vi "VXM Service modularLoop.vi"(6 "Standalone":bool=TRUE, 9 "Motion Cfg File path":path=path "C:/Users/Public/Documents/UCAR/APAR Board Test/SupportFiles/Motion64.ini", 10 "Cfg File path":path=path "C:/Users/Public/Documents/UCAR/APAR Board Test/SupportFiles/APARConfig.ini", 11 "MessageQues":T4) -> ()   [LabVIEW 2018]
doc: "This VI is a simple state machine that has a message que so it can be controlled by external processes.\nIt also has a control with all the messages ques in the calling application that it needs to send messages to.\n\nThe concept is to have many parallel VIs like this one. This VI should be a cohesive process. This could cut down on it's size and complexity.\n\nBolder Software LLC"
uses:
  Support/MessageQue/VXM Main Test App/MultipleMessageQues vxm.ctl
  Support/MessageQue/MessageQue.ctl
  Support/MessageQue/MessageCluster.ctl
  <instrlib>/Velmex VXM/Public/VXM Axis.ctl
  APARMainSubvis/VXM Public API/singleAxisMoveDef.ctl
  APARMainSubvis/VXM Public API/mmWaveAxis.ctl
  Classes/VXMCfg/VXMCfg.lvclass
  Classes/VXMMotionManager/VXMMotionManager.lvclass
  Classes/MotionComm/MotionComm.lvclass
  Classes/sub-systems/sub-systems.lvclass
  Classes/SendMessage/SendMessage.lvclass
  Support/MessageAPI/UIMessage.ctl
  Support/MessageQue/MessageQue.lvlib
  Classes/VSMx2/VXMx2.lvclass
  Classes/aparCfg/aparCfg.lvclass
  <instrlib>/Velmex VXM/Velmex VXM.lvlib
panel:
  out "Position":T1
  out "Axis (1..4)":T3=3 items=["X"=1, "Y"=2, "Z"=3, "T"=4]
  out "i":i32
  out "Command":string
  out "error out":errorcluster
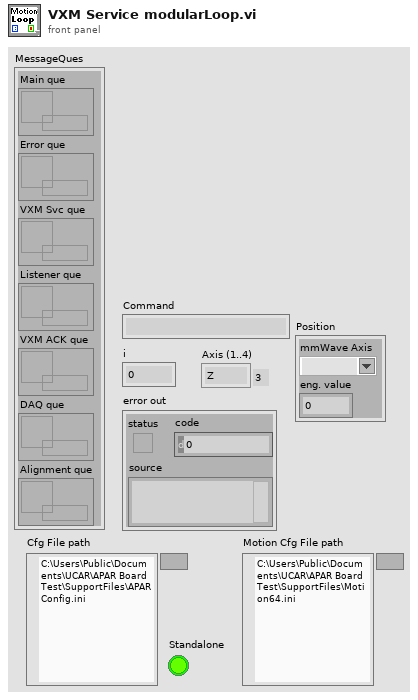
[diagram p1: front panel]
types:
  T1 = typedef "singleAxisMoveDef.ctl" = cluster{"mmWave Axis":T2, "eng. value":dbl}
  T2 = typedef "mmWaveAxis.ctl" = string
  T3 = typedef "Velmex VXM.lvlib/VXM Axis.ctl" = u16
  T4 = typedef "MultipleMessageQues vxm.ctl" = cluster{"Main que":T5, "Error que":T5, "VXM Svc que":T5, "Listener que":T5, "VXM ACK que":T5, "DAQ que":T5, "Alignment que":T5}
  T5 = typedef "MessageQue.lvlib/MessageQue.ctl" = refnum<queue>
  T6 = cluster{"VXMCfg":refnum<class "VXMCfg.lvclass">, "VXMMotionMGr":refnum<class "VXMMotionManager.lvclass">, "Motion":bool, "Motion ACK":refnum<class "MotionComm.lvclass">, "VXM Objects":refnum<class "sub-systems.lvclass">, "UIMsg":refnum<class "SendMessage.lvclass">}
  T7 = typedef "seqConfig.ctl" = cluster{"TempXMLFilePath":path, "Motion":bool}
  T8 = typedef "UIMessage.ctl" = cluster{"EventCode":i32, "Numeric":dbl, "String":string, "Variant":variant}
  T9 = cluster{"Subsystem 1, 2, 3":i32, "Set Home All subsystems":bool}
  T10 = cluster{"Move Type":string, "Positions":T1[], "Position (Antenna or Raster)":i32, "Polarization":u16}
  T11 = typedef "sub-syst.n.ctl" = cluster{"Addr":string, "Enable":bool, "X scale eng./step":dbl, "Y scale eng./step":dbl, "Z scale eng./step":dbl, "T scale eng./step":dbl, "X units":string, "Y units":string, "Z units":string, "T units":string, "X Jog":dbl, "Y Jog":dbl, "Z Jog":dbl, "T Jog":dbl, "X-1 Name":string, "Y-2 Name":string, "Z-3 Name":string, "T-4 Name":string, "VXM (1-4)":i32}
  T12 = cluster{"mmWaveName":string, "Sub-syst":i32, "Axis":string}[]
  T13 = cluster{"mmWave Names":string[], "Positions this subsystem":dbl[]}
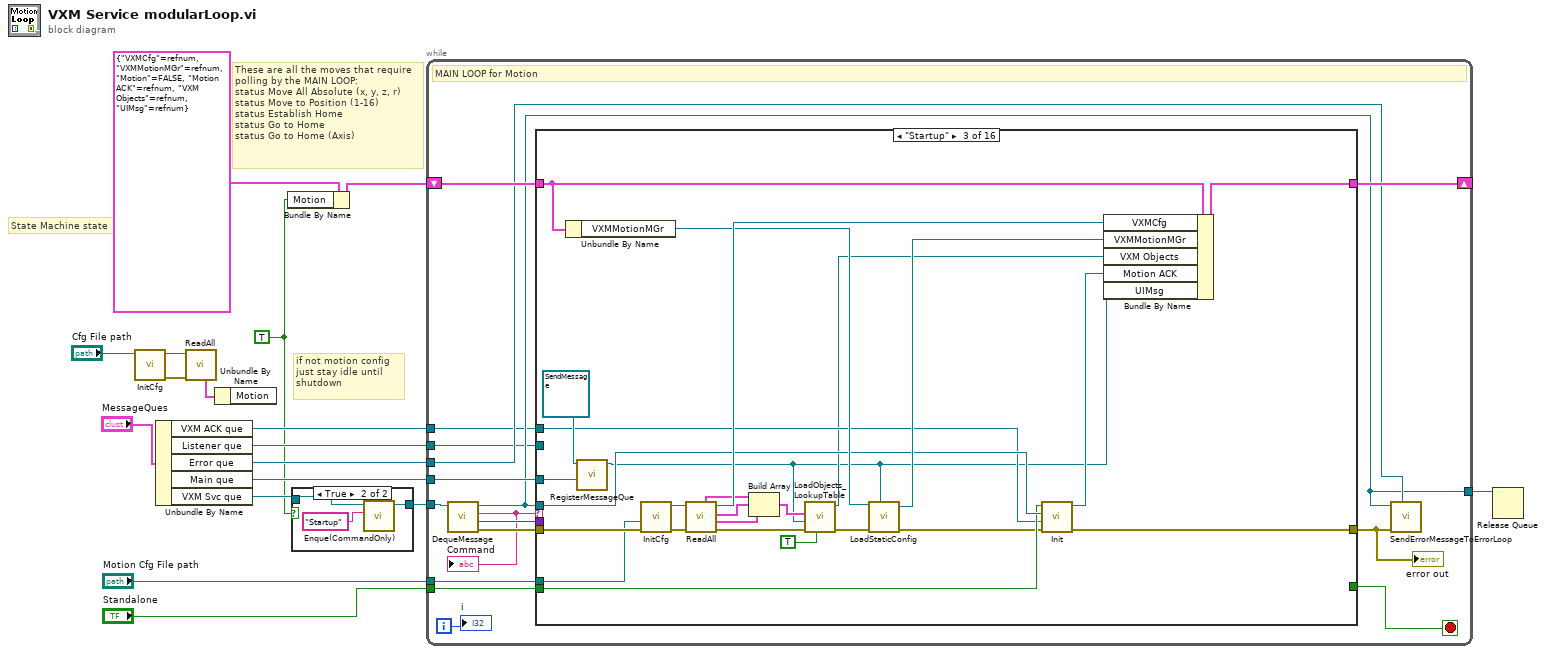
[diagram p0: block diagram]
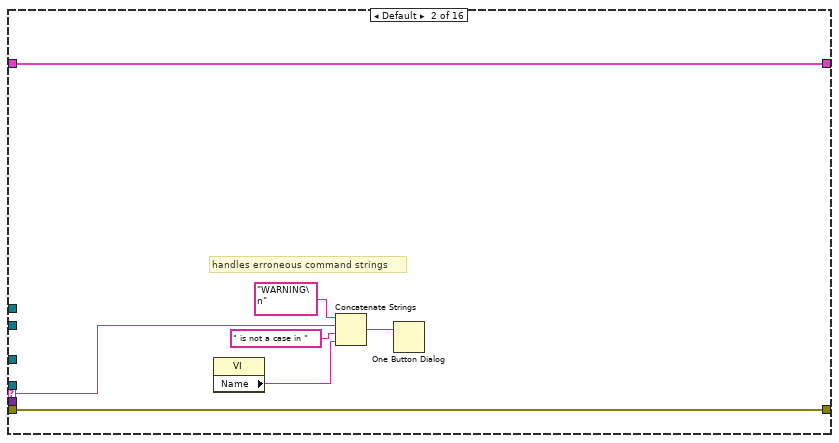
[diagram p4: hidden frame]
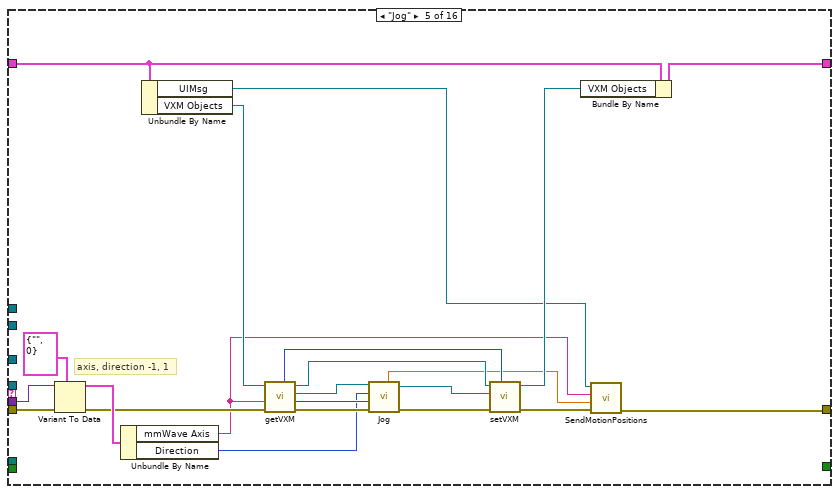
[diagram p6: hidden frame]
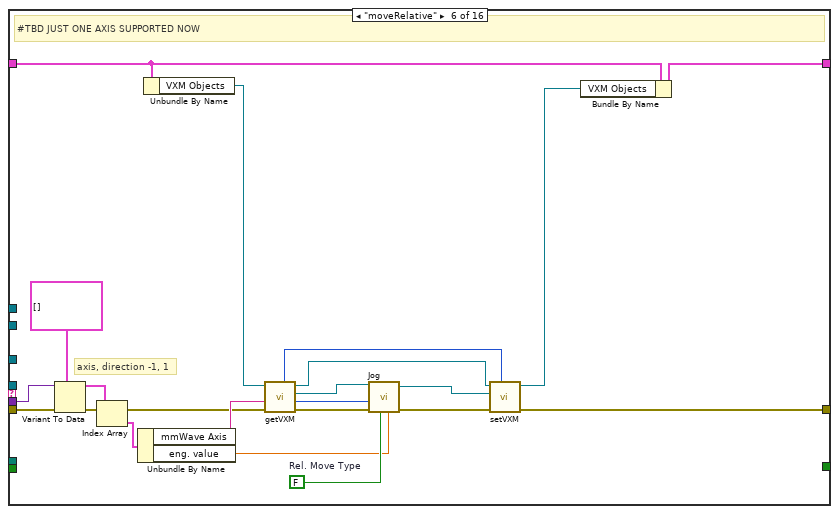
[diagram p7: hidden frame]
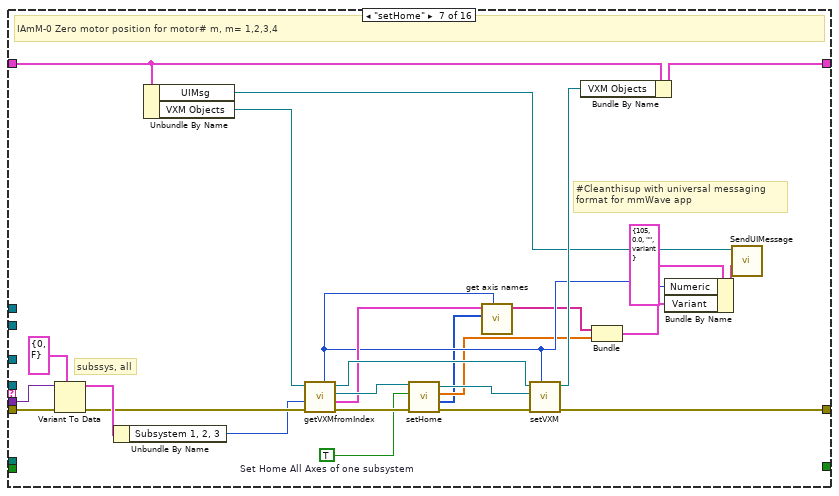
[diagram p8: hidden frame]
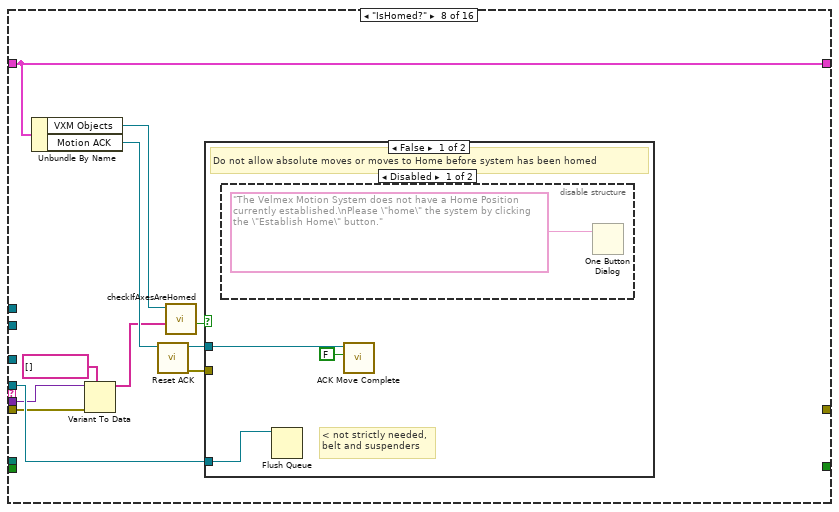
[diagram p9: hidden frame]
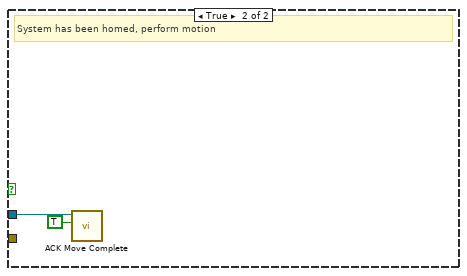
[diagram p11: hidden frame]
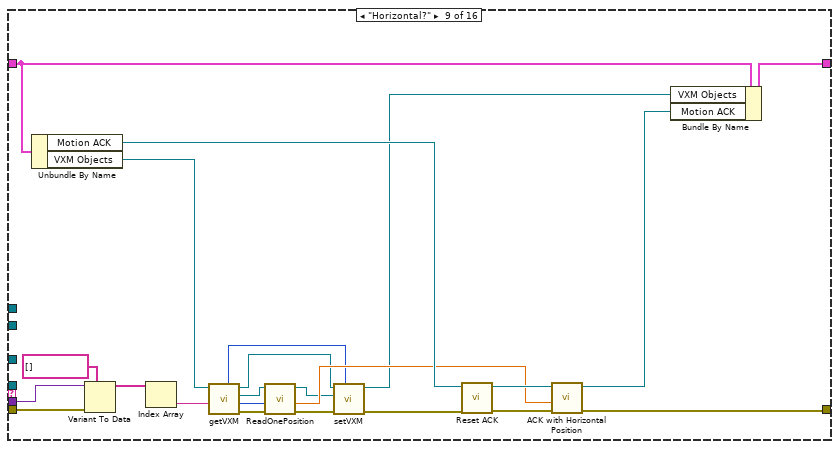
[diagram p12: hidden frame]
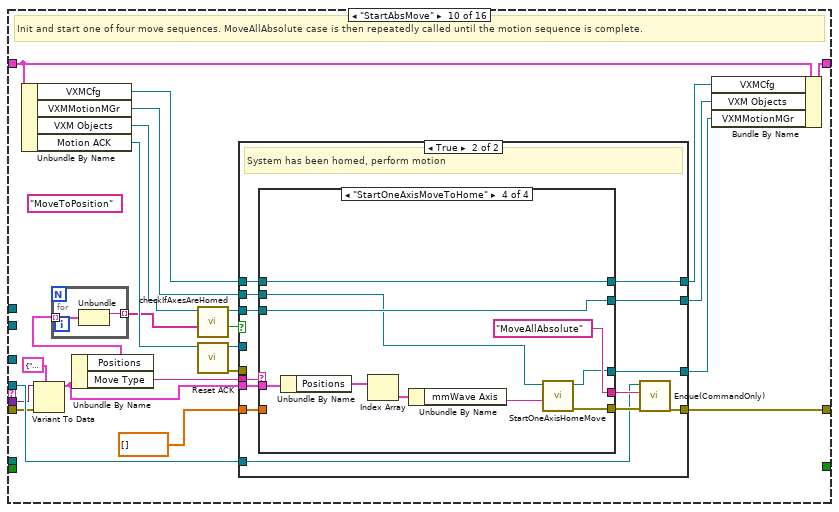
[diagram p13: hidden frame]
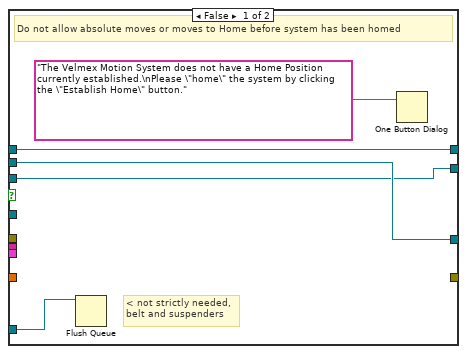
[diagram p14: hidden frame]
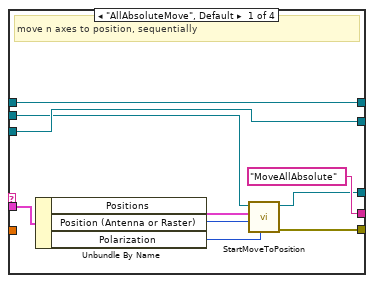
[diagram p15: hidden frame]
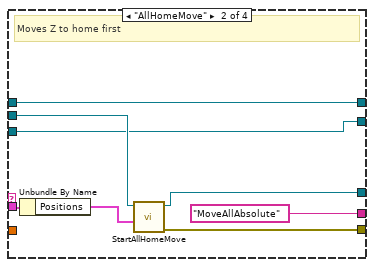
[diagram p16: hidden frame]
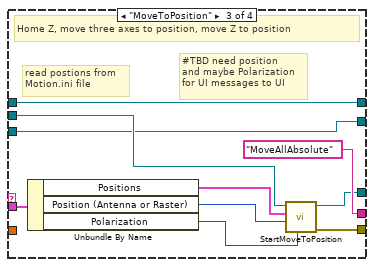
[diagram p17: hidden frame]
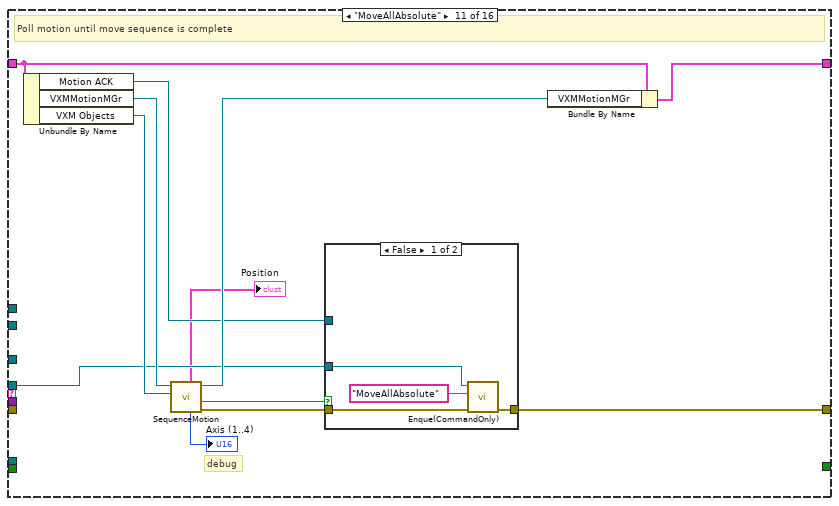
[diagram p18: hidden frame]
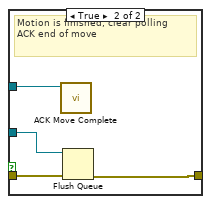
[diagram p19: hidden frame]
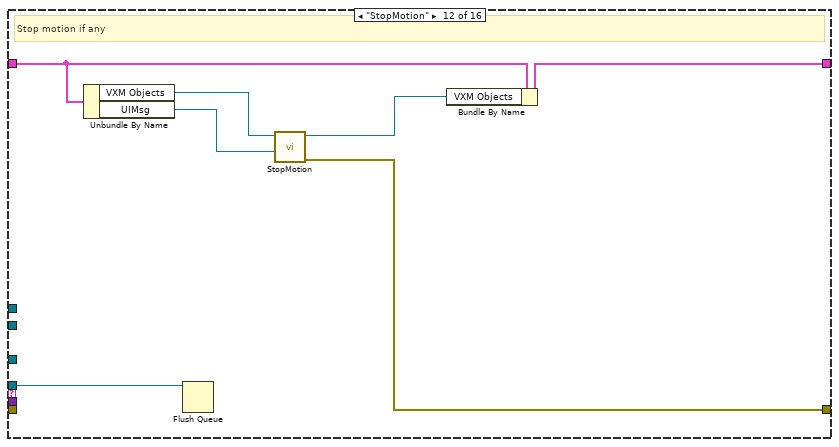
[diagram p20: hidden frame]
diagram:
  w1 = TRUE
  # "if not motion config\njust stay idle until\nshutdown"
  # "These are all the moves that require\npolling by the MAIN LOOP:\nstatus\tMove All Absolute (x, y, z, r)\nstatus\tMove to Position (1-16)\nstatus\tEstablish Home\nstatus\tGo to Home\nstatus\tGo to Home (Axis)"
  # "State Machine state"
  n1 = call "InitCfg.vi"("Cfg File path"="Cfg File path") -> ("error out"=w8:errorcluster, "aparCfg out"=w9:refnum<class "aparCfg.lvclass">)  [unwired: 9 in]
  n2 = Unbundle By Name("MessageQues") -> ("VXM ACK que"=w3:T5, "Listener que"=w11:T5, "Error que"=w15:T5, "Main que"=w16:T5, "VXM Svc que"=w13:T5)
  n3 = call "ReadAll.vi"("error in (no error)"=w8, "aparCfg in"=w9) -> ("SequenceConfig"=w6:T7)  [unwired: 4 in, 5 out]
  n4 = Unbundle By Name(w6) -> ()  [unwired: 1 out]
  n5 = Bundle By Name(cluster=T6 {"VXMCfg"=refnum, "VXMMotionMGr"=refnum, "Motion"=FALSE, "Motion ACK"=refnum, "VXM Objects"=refnum, "UIMsg"=refnum}, "Motion"=w1) -> (w5:T6)
  n6 = case shown="True" w1 {
    tunnel: w13 -> [w18 w21]
    tunnel: [w18 w20] -> w12
    frame False {
    }
    frame True {
      n7 = call "Enque(CommandOnly).vi"("Message Command"="Startup" ("Command"), "Message que"=w21) -> ("Message que out"=w20:T5)  [unwired: 8 in, 1 out]
    }
  }
  n8 = while {
    tunnel: w12 -> [w37]
    tunnel: w16 -> [w36]
    tunnel: w15 -> [w27]
    tunnel: [w26] -> w14
    shift-right: [w32] -> _
    shift-left: w5 -> [w31]
    tunnel: w11 -> [w25]
    tunnel: "Motion Cfg File path" -> [w24]
    tunnel: "Standalone" -> [w23]
    tunnel: w3 -> [w22]
    i -> [w30]
    stop <- w34 stop-if-true
    # "MAIN LOOP for Motion"
    n9 = call "DequeMessage.vi"("Message que"=w37) -> ("error out"=w35:errorcluster, "Message Payload"=w33:variant, "Message Command"=w29:string, "Message que out"=w26:T5)  [unwired: 5 in, 2 out]
    "Command" <- w29
    n10 = case shown="\"Startup\"" w29 {
      selector: w29 -> [_ w40 _ _ _ _ _ _ _ _ _ _ _ _ _ _]
      tunnel: w36 -> [_ _ w63 _ _ _ _ _ _ _ _ _ _ _ _ _]
      tunnel: w26 -> [_ _ w61 _ _ _ _ w147 _ w196 w265 w285 w288 _ _ _]
      tunnel: [_ w45 w47 _ w75 w112 w137 _ w170 w202 w268 w282 _ _ w296 _] -> w28
      tunnel: w35 -> [_ w45 w71 _ w83 w102 w130 w146 w177 w188 _ _ _ _ _ _]
      tunnel: [_ _ _ _ _ _ _ _ _ _ _ _ _ _ _ TRUE] -> w34
      tunnel: w33 -> [_ _ _ _ w82 w101 w129 w145 w176 w183 _ _ _ _ w295 _]
      tunnel: [w38 w44 w68 w72 w93 w113 w138 w143 w173 w200 w272 w286 w289 w293 w297 w301] -> w32
      tunnel: w31 -> [w38 w44 w66 w72 w94 w114 w139 w143 w174 w201 w261 w287 w289 w294 w297 w302]
      tunnel: w25 -> [_ _ _ _ _ _ _ _ _ _ _ _ _ _ _ _]
      tunnel: w24 -> [_ _ w48 _ _ _ _ _ _ _ _ _ _ _ _ _]
      tunnel: w23 -> [_ _ w60 _ _ _ _ _ _ _ _ _ _ _ _ _]
      tunnel: w22 -> [_ _ w59 _ _ _ _ _ _ _ _ _ _ _ _ _]
      frame "idle" {
      }
      frame Default {
        # "handles erroneous command strings"
        n11 = property class="VI"() -> ("Name"=w39:string)  [unwired: 2 in, 2 out]
        n12 = Concatenate Strings("WARNING\n" ("message"), w40, " is not a case in " ("message"), w39) -> (w43:string)
        n13 = One Button Dialog(message=w43) -> ()  [unwired: 1 in, 1 out]
      }
      frame "Startup" {
        n14 = Unbundle By Name(w66) -> ("VXMMotionMGr"=w65:refnum<class "VXMMotionManager.lvclass">)
        n15 = call "RegisterMessageQue.vi"("Message que"=w63, "SendMessage in"=refnum<class "SendMessage.lvclass"> refnum) -> ("SendMessage out"=w46:refnum<class "SendMessage.lvclass">)  [unwired: 8 in, 1 out]
        n16 = call "InitCfg.vi"("error in (no error)"=w71, "Cfg File path"=w48) -> ("error out"=w69:errorcluster, "VXMCfg out"=w70:refnum<class "VXMCfg.lvclass">)  [unwired: 7 in, 1 out]
        n17 = call "ReadAll.vi"("error in (no error)"=w69, "VXMCfg in"=w70) -> ("error out"=w56:errorcluster, "VXM Properties.sub-syst.3"=w53:T11, "VXM Properties.sub-syst.2"=w54:T11, "VXMCfg out"=w67:refnum<class "VXMCfg.lvclass">, "VXM Properties.sub-syst.1"=w55:T11)  [unwired: 5 in]
        n18 = Build Array(w55, w54, w53) -> (w52:T11[])
        n19 = call "LoadObjects_LookupTable.vi"("UIMsgReg."=TRUE, "error in (no error)"=w56, "UIMsg"=w46, "sub-system cfgs"=w52) -> ("error out"=w51:errorcluster, "sub-systems out"=w50:refnum<class "sub-systems.lvclass">)  [unwired: 6 in]
        n20 = call "LoadStaticConfig.vi"("UIMsg"=w46, "error in (no error)"=w51, "VXMMotionManager in"=w65) -> ("error out"=w57:errorcluster, "VXMMotionManager out"=w64:refnum<class "VXMMotionManager.lvclass">)  [unwired: 7 in]
        n21 = call "Init.vi"("error in (no error)"=w57, "VXM ACK que"=w59, "VXM Svc que"=w61, "Standalone"=w60) -> ("error out"=w47:errorcluster, "MotionComm out"=w58:refnum<class "MotionComm.lvclass">)  [unwired: 6 in]
        n22 = Bundle By Name(cluster=w66, "VXMCfg"=w67, "VXMMotionMGr"=w64, "VXM Objects"=w50, "Motion ACK"=w58, "UIMsg"=w46) -> (w68:T6)
      }
      frame "UpdateJogProperties" {
      }
      frame "Jog" {
        # "axis, direction -1, 1"
        n23 = Variant To Data(error in=w83, type=cluster{"mmWave Axis":T2, "Direction":i32} {"mmWave Axis"="", "Direction"=0} ("output cluster"), Variant=w82) -> (data=w91:cluster{"mmWave Axis":T2, "Direction":i32}, error out=w81:errorcluster)
        n24 = Unbundle By Name(w91) -> ("mmWave Axis"=w73:T2, "Direction"=w79:i32)
        n25 = Unbundle By Name(w94) -> ("UIMsg"=w74:refnum<class "SendMessage.lvclass">, "VXM Objects"=w88:refnum<class "sub-systems.lvclass">)
        n26 = call "getVXM.vi"("error in (no error)"=w81, "mmWave Axis Name"=w73, "sub-systems in"=w88) -> ("error out"=w80:errorcluster, "Axis (1..4)"=w84:T3, "VXMx2 out"=w86:refnum<class "VXMx2.lvclass">, "sub-systems out"=w87:refnum<class "sub-systems.lvclass">, "Sub-syst number"=w85:i32)  [unwired: 4 in]
        n27 = call "Jog.vi"("error in (no error)"=w80, "Axis (1..4)"=w84, "Direction -1, 1"=w79, "VXMx2 in"=w86) -> ("error out"=w77:errorcluster, "VXMx2 out"=w89:refnum<class "VXMx2.lvclass">, "Position, eng units"=w78:dbl)  [unwired: 5 in]
        n28 = call "setVXM.vi"("Sub-syst number"=w85, "error in (no error)"=w77, "VXMn"=w89, "sub-systems in"=w87) -> ("error out"=w76:errorcluster, "sub-systems out"=w90:refnum<class "sub-systems.lvclass">)  [unwired: 6 in]
        n29 = Bundle By Name(cluster=w94, "VXM Objects"=w90) -> (w93:T6)
        n30 = call "SendMotionPositions.vi"("error in (no error)"=w76, "Axis Position, eng."=w78, "mmWave Axis Name"=w73, "SendMessage in"=w74) -> ("error out"=w75:errorcluster)  [unwired: 6 in, 1 out]
      }
      frame "moveRelative" {
        w98 = FALSE  # Rel. Move Type
        # "axis, direction -1, 1"
        # "#TBD JUST ONE AXIS SUPPORTED NOW"
        n31 = Variant To Data(error in=w102, type=T1[] [] ("Moves"), Variant=w101) -> (data=w111:T1[], error out=w100:errorcluster)
        n32 = Index Array(array=w111) -> (element=w95:T1)  [unwired: 1 in]
        n33 = Unbundle By Name(w95) -> ("mmWave Axis"=w108:T2, "eng. value"=w97:dbl)
        n34 = Unbundle By Name(w114) -> ("VXM Objects"=w107:refnum<class "sub-systems.lvclass">)
        n35 = call "getVXM.vi"("error in (no error)"=w100, "mmWave Axis Name"=w108, "sub-systems in"=w107) -> ("error out"=w99:errorcluster, "Axis (1..4)"=w103:T3, "VXMx2 out"=w105:refnum<class "VXMx2.lvclass">, "sub-systems out"=w106:refnum<class "sub-systems.lvclass">, "Sub-syst number"=w104:i32)  [unwired: 4 in]
        n36 = call "Jog.vi"("One Axis Rel Distanz mm"=w97, "Rel. Move Type"=w98, "error in (no error)"=w99, "Axis (1..4)"=w103, "VXMx2 in"=w105) -> ("error out"=w112:errorcluster, "VXMx2 out"=w109:refnum<class "VXMx2.lvclass">)  [unwired: 4 in, 1 out]
        n37 = call "setVXM.vi"("Sub-syst number"=w104, "VXMn"=w109, "sub-systems in"=w106) -> ("sub-systems out"=w110:refnum<class "sub-systems.lvclass">)  [unwired: 7 in, 1 out]
        n38 = Bundle By Name(cluster=w114, "VXM Objects"=w110) -> (w113:T6)
      }
      frame "setHome" {
        w124 = TRUE  # Set Home All Axes of one subsystem
        # "#Cleanthisup with universal messaging \nformat for mmWave app"
        # "subssys, all"
        # "IAmM-0 Zero motor position for motor# m, m= 1,2,3,4"
        n39 = Variant To Data(error in=w130, type=T9 {"Subsystem 1, 2, 3"=0, "Set Home All subsystems"=FALSE} ("output cluster"), Variant=w129) -> (data=w136:T9, error out=w128:errorcluster)
        n40 = Unbundle By Name(w136) -> ("Subsystem 1, 2, 3"=w125:i32)
        n41 = Unbundle By Name(w139) -> ("UIMsg"=w121:refnum<class "SendMessage.lvclass">, "VXM Objects"=w133:refnum<class "sub-systems.lvclass">)
        n42 = call "getVXMfromIndex.vi"("error in (no error)"=w128, "Subsystem 1, 2, 3"=w125, "sub-systems in"=w133) -> ("error out"=w127:errorcluster, "All Axes this subsystem"=w120:T12, "VXMx2 out"=w131:refnum<class "VXMx2.lvclass">, "sub-systems out"=w132:refnum<class "sub-systems.lvclass">, "Sub-syst number"=w119:i32)  [unwired: 4 in]
        n43 = call "setHome.vi"("error in (no error)"=w127, "Set Home All Axes"=w124, "VXMx2 in"=w131) -> ("error out"=w137:errorcluster, "Axes"=w115:T3[], "Positions this subsystem"=w117:dbl[], "VXMx2 out"=w134:refnum<class "VXMx2.lvclass">)  [unwired: 5 in]
        n44 = call "get axis names.vi"("Subsystem 1, 2, 3"=w119, "Axes"=w115, "Lookup Table"=w120) -> ("mmWave Names"=w118:string[])  [unwired: 8 in]
        n45 = call "setVXM.vi"("Sub-syst number"=w119, "VXMn"=w134, "sub-systems in"=w132) -> ("sub-systems out"=w135:refnum<class "sub-systems.lvclass">)  [unwired: 7 in, 1 out]
        n46 = Bundle By Name(cluster=w139, "VXM Objects"=w135) -> (w138:T6)
        n47 = Bundle("mmWave Names"=w118, "Positions this subsystem"=w117) -> (w116:T13)  [unwired: 1 in]
        n48 = Bundle By Name(cluster=T8 {"EventCode"=105, "Numeric"=0.0, "String"="", "Variant"=variant} ("UIMsg"), "Numeric"=w119, "Variant"=w116) -> (w122:T8)
        n49 = call-dynamic "SendUIMessage.vi"("UIMsg"=w122, "SendMessage in"=w121) -> ()  [unwired: 8 in, 2 out]
      }
      frame "IsHomed?" {
        n50 = Unbundle By Name(w143) -> ("VXM Objects"=w142:refnum<class "sub-systems.lvclass">, "Motion ACK"=w150:refnum<class "MotionComm.lvclass">)
        n51 = Variant To Data(error in=w146, type=T2[] [] ("check these axes homed"), Variant=w145) -> (data=w141:T2[])  [unwired: 1 out]
        n52 = call "Reset ACK.vi"("MotionComm in"=w150) -> ("error out"=w149:errorcluster, "MotionComm out"=w148:refnum<class "MotionComm.lvclass">)  [unwired: 9 in]
        n53 = call "checkIfAxesAreHomed.vi"("check these axes homed"=w141, "sub-systems in"=w142) -> ("Homed=T"=w140:bool)  [unwired: 7 in, 2 out]
        n54 = case shown="False" w140 {
          tunnel: w147 -> [w153 _]
          tunnel: w149 -> [_ _]
          tunnel: w148 -> [w152 w155]
          frame False {
            # "< not strictly needed,\nbelt and suspenders"
            # "Do not allow absolute moves or moves to Home before system has been homed"
            n55 = disable-structure shown="Disabled" {
              frame Disabled {
                n56 = One Button Dialog(message="The Velmex Motion System does not have a Home Position currently established.\nPlease \"home\" the system by clicking the \"Establish Home\" button.") -> ()  [unwired: 1 in, 1 out]
              }
              frame Enabled {
              }
            }
            n57 = Flush Queue(queue=w153) -> ()  [unwired: 1 in, 3 out]
            n58 = call "ACK Move Complete.vi"("Motion ACK = True"=FALSE, "MotionComm in"=w152) -> ()  [unwired: 8 in, 2 out]
          }
          frame True {
            # "System has been homed, perform motion"
            n59 = call "ACK Move Complete.vi"("Motion ACK = True"=TRUE, "MotionComm in"=w155) -> ()  [unwired: 8 in, 2 out]
          }
        }
      }
      frame "Horizontal?" {
        n60 = Unbundle By Name(w174) -> ("Motion ACK"=w179:refnum<class "MotionComm.lvclass">, "VXM Objects"=w168:refnum<class "sub-systems.lvclass">)
        n61 = Variant To Data(error in=w177, type=T2[] [] ("check these axes homed"), Variant=w176) -> (data=w169:T2[])  [unwired: 1 out]
        n62 = Index Array(array=w169) -> (element=w167:T2)  [unwired: 1 in]
        n63 = call "getVXM.vi"("mmWave Axis Name"=w167, "sub-systems in"=w168) -> ("error out"=w166:errorcluster, "Axis (1..4)"=w164:T3, "VXMx2 out"=w165:refnum<class "VXMx2.lvclass">, "sub-systems out"=w159:refnum<class "sub-systems.lvclass">, "Sub-syst number"=w160:i32)  [unwired: 5 in]
        n64 = call "ReadOnePosition.vi"("error in (no error)"=w166, "Axis (1..4)"=w164, "VXMx2 in"=w165) -> ("error out"=w162:errorcluster, "Position, eng units"=w163:dbl, "VXMx2 out"=w158:refnum<class "VXMx2.lvclass">)  [unwired: 6 in]
        n65 = call "setVXM.vi"("Sub-syst number"=w160, "error in (no error)"=w162, "VXMn"=w158, "sub-systems in"=w159) -> ("error out"=w161:errorcluster, "sub-systems out"=w157:refnum<class "sub-systems.lvclass">)  [unwired: 6 in]
        n66 = call "Reset ACK.vi"("error in (no error)"=w161, "MotionComm in"=w179) -> ("error out"=w171:errorcluster, "MotionComm out"=w178:refnum<class "MotionComm.lvclass">)  [unwired: 8 in]
        n67 = call "ACK with Horizontal Position.vi"("error in (no error)"=w171, "Horizontal position, degrees"=w163, "MotionComm in"=w178) -> ("error out"=w170:errorcluster, "MotionComm out"=w172:refnum<class "MotionComm.lvclass">)  [unwired: 7 in]
        n68 = Bundle By Name(cluster=w174, "VXM Objects"=w157, "Motion ACK"=w172) -> (w173:T6)
      }
      frame "StartAbsMove" {
        (unwired) "MoveToPosition" ("MoveType")
        # "Init and start one of four move sequences. MoveAllAbsolute case is then repeatedly called until the motion sequence is complete."
        n69 = Unbundle By Name(w201) -> ("VXMCfg"=w195:refnum<class "VXMCfg.lvclass">, "VXMMotionMGr"=w199:refnum<class "VXMMotionManager.lvclass">, "VXM Objects"=w180:refnum<class "sub-systems.lvclass">, "Motion ACK"=w193:refnum<class "MotionComm.lvclass">)
        n70 = Variant To Data(error in=w188, type=T10 {"Move Type"="OneAxisHomeMove", "Positions"=[], "Position (Antenna or Raster)"=0, "Polarization"=0} ("Move-Abs"), Variant=w183) -> (data=w185:T10)  [unwired: 1 out]
        n71 = Unbundle By Name(w185) -> ("Positions"=w182:T1[], "Move Type"=w186:string)
        n72 = for {
          tunnel: w182 -> [w204] mode=indexing
          tunnel: [w203] -> w181 mode=indexing
          n73 = Unbundle(w204) -> ("mmWave Axis"=w203:T2)  [unwired: 1 out]
        }
        n74 = call "checkIfAxesAreHomed.vi"("check these axes homed"=w181, "sub-systems in"=w180) -> ("Homed=T"=w189:bool, "sub-systems out"=w190:refnum<class "sub-systems.lvclass">)  [unwired: 7 in, 1 out]
        n75 = call "Reset ACK.vi"("MotionComm in"=w193) -> ("error out"=w192:errorcluster, "MotionComm out"=w191:refnum<class "MotionComm.lvclass">)  [unwired: 9 in]
        n76 = case shown="True" w189 {
          tunnel: [_ w222] -> w202
          tunnel: w186 -> [_ w221]
          tunnel: w199 -> [w209 w220]
          tunnel: dbl[] [] ("Move Params") -> [_ w219]
          tunnel: [w209 w216] -> w197
          tunnel: w190 -> [w205 w215]
          tunnel: w196 -> [w207 w214]
          tunnel: w195 -> [w206 w213]
          tunnel: [w206 w212] -> w194
          tunnel: w192 -> [_ _]
          tunnel: w191 -> [_ _]
          tunnel: w185 -> [_ w211]
          tunnel: [w205 w210] -> w187
          frame False {
            # "< not strictly needed,\nbelt and suspenders"
            # "Do not allow absolute moves or moves to Home before system has been homed"
            n77 = Flush Queue(queue=w207) -> ()  [unwired: 1 in, 3 out]
            n78 = One Button Dialog(message="The Velmex Motion System does not have a Home Position currently established.\nPlease \"home\" the system by clicking the \"Establish Home\" button.") -> ()  [unwired: 1 in, 1 out]
          }
          frame True {
            # "System has been homed, perform motion"
            n79 = case shown="\"StartOneAxisMoveToHome\"" w221 {
              tunnel: w220 -> [w226 w240 w246 w254]
              tunnel: w219 -> [_ _ _ _]
              tunnel: ["MoveAllAbsolute" ("Command") "MoveAllAbsolute" ("Command") "MoveAllAbsolute" ("Command") "MoveAllAbsolute" ("Command")] -> w218
              tunnel: [w229 w238 w249 w256] -> w217
              tunnel: w215 -> [w230 w235 w245 w258]
              tunnel: [w228 w237 w248 w255] -> w216
              tunnel: w213 -> [w231 w236 w247 w259]
              tunnel: [w231 w236 w247 w259] -> w212
              tunnel: w211 -> [w227 w234 w244 w257]
              tunnel: [w230 w235 w245 w258] -> w210
              frame "AllAbsoluteMove", Default {
                # "move n axes to position, sequentially"
                n80 = Unbundle By Name(w227) -> ("Positions"=w223:T1[], "Position (Antenna or Raster)"=w225:i32, "Polarization"=w224:u16)
                n81 = call "StartMoveToPosition.vi"("Polarization"=w224, "Position (Antenna or Raster)"=w225, "Positions"=w223, "VXMMotionManager in"=w226) -> ("error out"=w229:errorcluster, "VXMMotionManager out"=w228:refnum<class "VXMMotionManager.lvclass">)  [unwired: 6 in]
              }
              frame "AllHomeMove" {
                # "Moves Z to home first"
                n82 = Unbundle By Name(w234) -> ("Positions"=w233:T1[])
                n83 = call "StartAllHomeMove.vi"("Positions to home"=w233, "VXMMotionManager in"=w240) -> ("error out"=w238:errorcluster, "VXMMotionManager out"=w237:refnum<class "VXMMotionManager.lvclass">)  [unwired: 8 in]
              }
              frame "MoveToPosition" {
                # "#TBD need position\nand maybe Polarization\nfor UI messages to UI"
                # "read postions from \nMotion.ini file"
                # "Home Z, move three axes to position, move Z to position"
                n84 = Unbundle By Name(w244) -> ("Positions"=w243:T1[], "Position (Antenna or Raster)"=w242:i32, "Polarization"=w241:u16)
                n85 = call "StartMoveToPosition.vi"("Polarization"=w241, "Position (Antenna or Raster)"=w242, "Positions"=w243, "VXMMotionManager in"=w246) -> ("error out"=w249:errorcluster, "VXMMotionManager out"=w248:refnum<class "VXMMotionManager.lvclass">)  [unwired: 6 in]
              }
              frame "StartOneAxisMoveToHome" {
                n86 = Unbundle By Name(w257) -> ("Positions"=w253:T1[])
                n87 = Index Array(array=w253) -> (element=w252:T1)  [unwired: 1 in]
                n88 = Unbundle By Name(w252) -> ("mmWave Axis"=w251:T2)
                n89 = call "StartOneAxisHomeMove.vi"("mmWave Axis to Home"=w251, "VXMMotionManager in"=w254) -> ("error out"=w256:errorcluster, "VXMMotionManager out"=w255:refnum<class "VXMMotionManager.lvclass">)  [unwired: 8 in]
              }
            }
            n90 = call "Enque(CommandOnly).vi"("error in"=w217, "Message Command"=w218, "Message que"=w214) -> ("error out"=w222:errorcluster)  [unwired: 7 in, 1 out]
          }
        }
        n91 = Bundle By Name(cluster=w201, "VXMCfg"=w194, "VXM Objects"=w187, "VXMMotionMGr"=w197) -> (w200:T6)
      }
      frame "MoveAllAbsolute" {
        # "debug"
        # "Poll motion until move sequence is complete"
        n92 = Unbundle By Name(w261) -> ("Motion ACK"=w263:refnum<class "MotionComm.lvclass">, "VXMMotionMGr"=w271:refnum<class "VXMMotionManager.lvclass">, "VXM Objects"=w269:refnum<class "sub-systems.lvclass">)
        n93 = call "SequenceMotion.vi"("sub-systems in"=w269, "VXMMotionManager in"=w271) -> ("error out"=w267:errorcluster, "Motions Finished = T"=w266:bool, "VXMMotionManager out"=w270:refnum<class "VXMMotionManager.lvclass">, "Axis Number"=→"Axis (1..4)":i32, "Position"=→"Position":T1)  [unwired: 4 in, 1 out]
        n94 = case shown="False" w266 {
          tunnel: [w275 w279] -> w268
          tunnel: w267 -> [w274 w280]
          tunnel: w265 -> [w273 w278]
          tunnel: w263 -> [_ w277]
          frame False {
            n95 = call "Enque(CommandOnly).vi"("error in"=w274, "Message Command"="MoveAllAbsolute" ("Command"), "Message que"=w273) -> ("error out"=w275:errorcluster)  [unwired: 7 in, 1 out]
          }
          frame True {
            # "Motion is finished, clear polling\nACK end of move"
            n96 = call "ACK Move Complete.vi"("MotionComm in"=w277) -> ()  [unwired: 9 in, 2 out]
            n97 = Flush Queue(queue=w278, error in (no error)=w280) -> (error out=w279:errorcluster)  [unwired: 2 out]
          }
        }
        n98 = Bundle By Name(cluster=w261, "VXMMotionMGr"=w270) -> (w272:T6)
      }
      frame "StopMotion" {
        # "Stop motion if any"
        n99 = Unbundle By Name(w287) -> ("VXM Objects"=w284:refnum<class "sub-systems.lvclass">, "UIMsg"=w281:refnum<class "SendMessage.lvclass">)
        n100 = Flush Queue(queue=w285) -> ()  [unwired: 1 in, 3 out]
        n101 = call "StopMotion.vi"("SendMessage"=w281, "sub-systems in"=w284) -> ("error out"=w282:errorcluster, "sub-systems out"=w283:refnum<class "sub-systems.lvclass">)  [unwired: 8 in]
        n102 = Bundle By Name(cluster=w287, "VXM Objects"=w283) -> (w286:T6)
      }
      frame "Flush" {
        n103 = Flush Queue(queue=w288) -> ()  [unwired: 1 in, 3 out]
      }
      frame "Stop_Close" {
        # "ignore errors"
        n104 = Unbundle By Name(w294) -> ("VXM Objects"=w291:refnum<class "sub-systems.lvclass">)
        n105 = call "CloseAll.vi"("sub-systems in"=w291) -> ("error out"=w292:errorcluster, "sub-systems out"=w290:refnum<class "sub-systems.lvclass">)  [unwired: 9 in]
        n106 = flat-sequence {
          tunnel: w292 -> [_]
          frame #0 {
          }
        }
        n107 = Bundle By Name(cluster=w294, "VXM Objects"=w290) -> (w293:T6)
      }
      frame "GenerateTestError" {
        n108 = call "ConvertTo(error).vi"("Message Payload"=w295) -> ("Message Payload error"=w296:errorcluster)  [unwired: 9 in, 1 out]
      }
      frame "ExitNow" {
        # "ignore errors"
        n109 = Unbundle By Name(w302) -> ("VXM Objects"=w300:refnum<class "sub-systems.lvclass">)
        n110 = call "CloseAll.vi"("sub-systems in"=w300) -> ("error out"=w298:errorcluster, "sub-systems out"=w299:refnum<class "sub-systems.lvclass">)  [unwired: 9 in]
        n111 = flat-sequence {
          tunnel: w298 -> [_]
          frame #0 {
          }
        }
        n112 = Bundle By Name(cluster=w302, "VXM Objects"=w299) -> (w301:T6)
      }
    }
    "error out" <- w28
    n113 = call "SendErrorMessageToErrorLoop.vi"("Error Message que"=w27, "error in (no error)"=w28, "Loop Message que"=w26) -> ()  [unwired: 8 in, 1 out]
    "i" <- w30
  }
  n114 = Release Queue(queue=w14) -> ()  [unwired: 2 in, 3 out]
